vi "Write Open_Close.vi"(8 "error in (no error)":errorcluster, 10 "Open/Close":bool, 11 "PacMan in":refnum<class "PacMan.lvclass">) -> (0 "error out":errorcluster, 3 "PacMan out":refnum<class "PacMan.lvclass">)   [LabVIEW 2016, in "PacManClasses.lvlib" / "PacMan.lvclass"]
uses:
  PacMan.lvclass
  PacMan.lvclass/PacMan.ctl
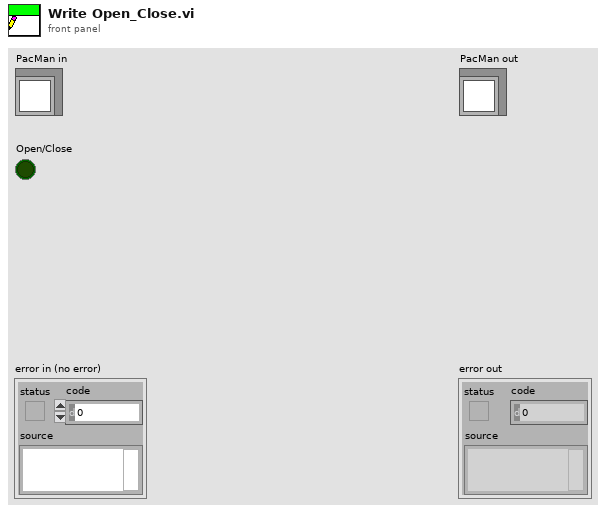
[diagram p1: front panel]
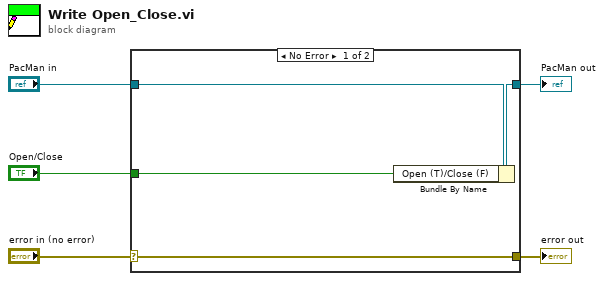
[diagram p0: block diagram]
diagram:
  n1 = case shown="No Error" "error in (no error)" {
    selector: "error in (no error)" -> [w9 w10]
    tunnel: [w9 w10] -> w4
    tunnel: [w7 w11] -> w2
    tunnel: "PacMan in" -> [w8 w11]
    tunnel: "Open/Close" -> [w6 _]
    frame No Error {
      n2 = Bundle By Name(cluster=w8, "Open (T)/Close (F)"=w6) -> (w7:refnum<class "PacMan.lvclass">)
    }
    frame Error {
    }
  }
  "error out" <- w4
  "PacMan out" <- w2
